vi "ParseGetRequest.vi"(11 "body":string) -> (2 "result string":string, 3 "Array":string[][](array[string]))   [LabVIEW 2015]
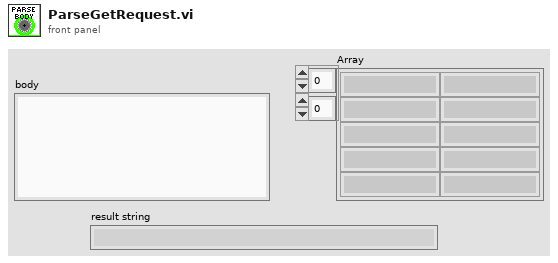
[diagram p1: front panel]
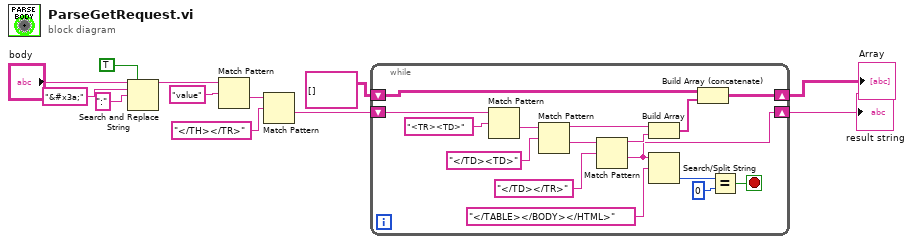
[diagram p0: block diagram]
diagram:
  n1 = Search and Replace String(replace all?=TRUE ("replace all? (F)"), input string="body", search string="&#x3a;", replace string=":" ("replace string (\"\")")) -> (result string=w3:string)  [unwired: 4 in, 3 out]
  n2 = Match Pattern(string=w3, regular expression="value") -> (after substring=w9:string)  [unwired: 1 in, 3 out]
  n3 = Match Pattern(string=w9, regular expression="</TH></TR>") -> (after substring=w7:string)  [unwired: 1 in, 3 out]
  n4 = while {
    shift-right: [w17] -> w5
    shift-left: w7 -> [w14]
    shift-right: [w18] -> w6
    shift-left: string[][] [] -> [w28]
    stop <- w16 stop-if-true
    n5 = Match Pattern(string=w14, regular expression="<TR><TD>") -> (after substring=w13:string)  [unwired: 1 in, 3 out]
    n6 = Match Pattern(string=w13, regular expression="</TD><TD>") -> (before substring=w26:string, after substring=w20:string)  [unwired: 1 in, 2 out]
    n7 = Match Pattern(string=w20, regular expression="</TD></TR>") -> (before substring=w19:string, after substring=w17:string)  [unwired: 1 in, 2 out]
    n8 = Build Array(w26, w19) -> (w25:string[])
    n9 = Search/Split String(string=w17, search string/char (-)="</TABLE></BODY></HTML>" ("true string")) -> (offset of match=w23:i32)  [unwired: 1 in, 2 out]
    n10 = Build Array (concatenate)(w28, w25) -> (w18:string[][])
    n11 = Equal?(x=w23, y=0) -> (x = y?=w16:bool)
  }
  "Array" <- w6
  "result string" <- w5
